vi "S101_temp_rise_red.vi"(0 "SI101_AverageReactorCoolantTemperature.lvclass":refnum<class "SI101_AverageReactorCoolantTemperature.lvclass">, 1 "3 JEC10 CT001B XQ01":dbl, 2 "3 JEC20 CT001B XQ01":dbl, 3 "3 JEC30 CT001B XQ01":dbl, 4 "3 JEC40 CT001B XQ01":dbl, 5 "error in (no error)":errorcluster, 6 "From Acquisition":T3, 8 "From SI100":T2) -> (12 "APs":cluster{"AP1":dbl, "AP2":dbl, "AP3":dbl}, 14 "SI101_AverageReactorCoolantTemperature.lvclass out":refnum<class "SI101_AverageReactorCoolantTemperature.lvclass">, 15 "ACT Loop 1":dbl, 16 "ACT Loop 2":dbl, 17 "ACT loop 3":dbl, 18 "ACT loop 4":dbl, 19 "error IO":errorcluster)   [LabVIEW 2022 SP3, in "SI101_AverageReactorCoolantTemperature.lvclass"]
uses:
  SI101_AverageReactorCoolantTemperature.lvclass
  SI101_AverageReactorCoolantTemperature.lvclass/SI101_AverageReactorCoolantTemperature.ctl
panel:
  in  "Set Params 4":T1
  in  "Set Params 3":T1
  in  "Set Params 2":T1
  in  "Set Params":T1
  # "SI101"
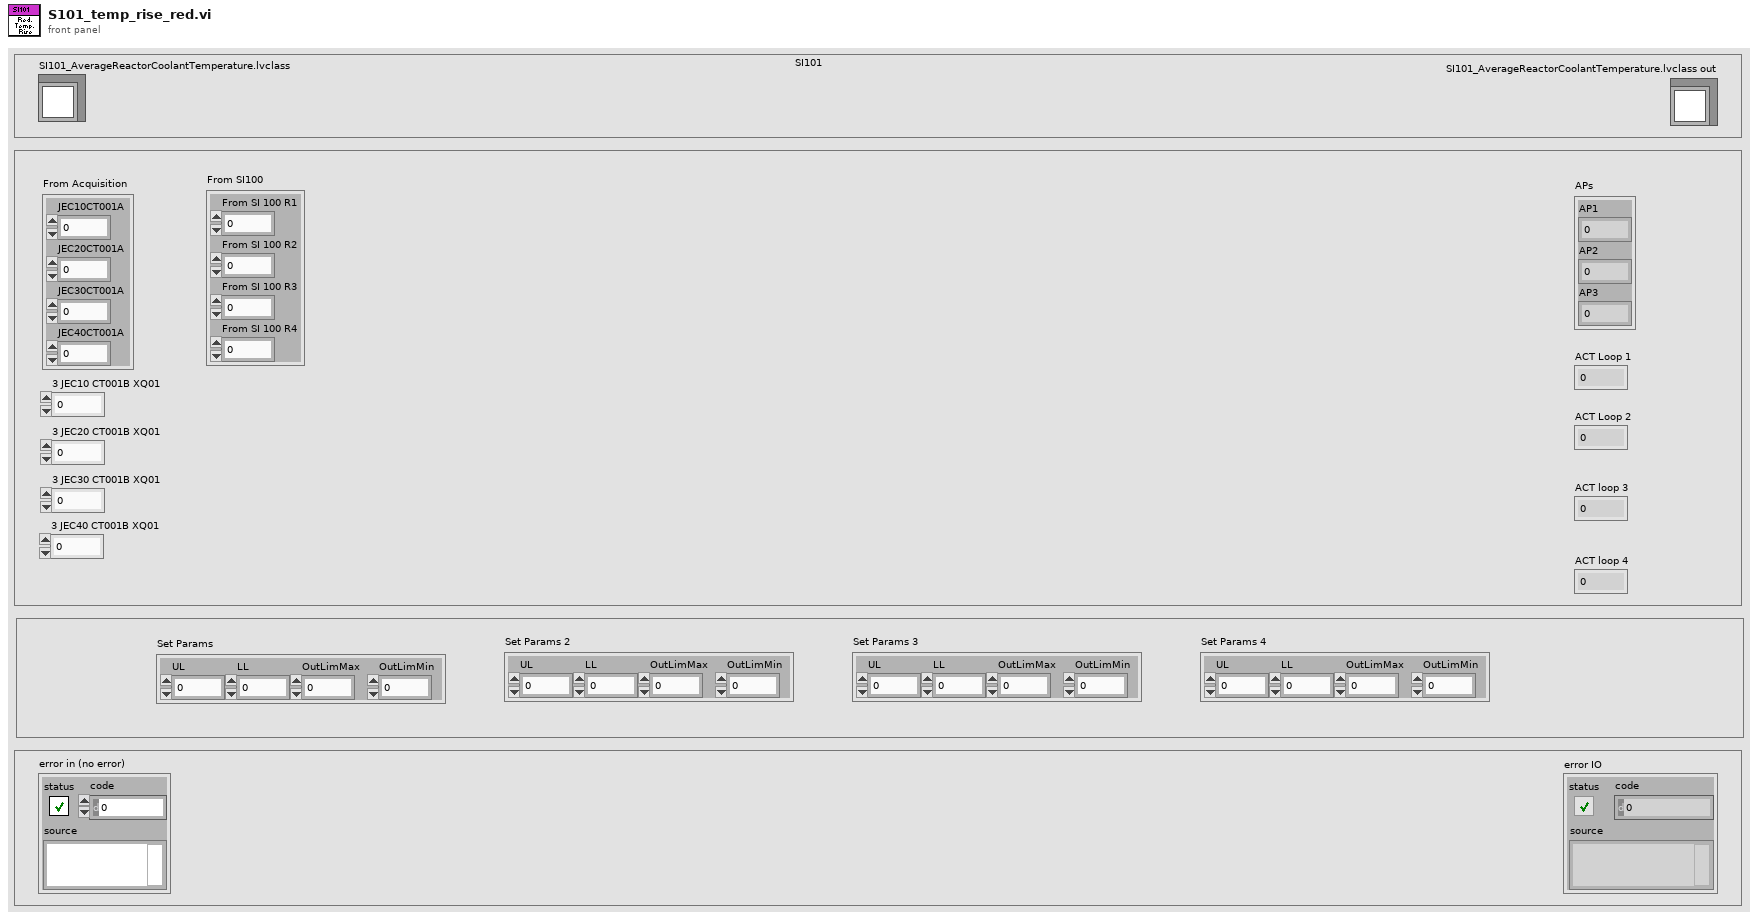
[diagram p1: front panel]
types:
  T1 = cluster{"UL":dbl, "LL":dbl, "OutLimMax":dbl, "OutLimMin":dbl}
  T2 = cluster{"From SI 100 R1":dbl, "From SI 100 R2":dbl, "From SI 100 R3":dbl, "From SI 100 R4":dbl}
  T3 = cluster{"JEC10CT001A":dbl, "JEC20CT001A":dbl, "JEC30CT001A":dbl, "JEC40CT001A":dbl}
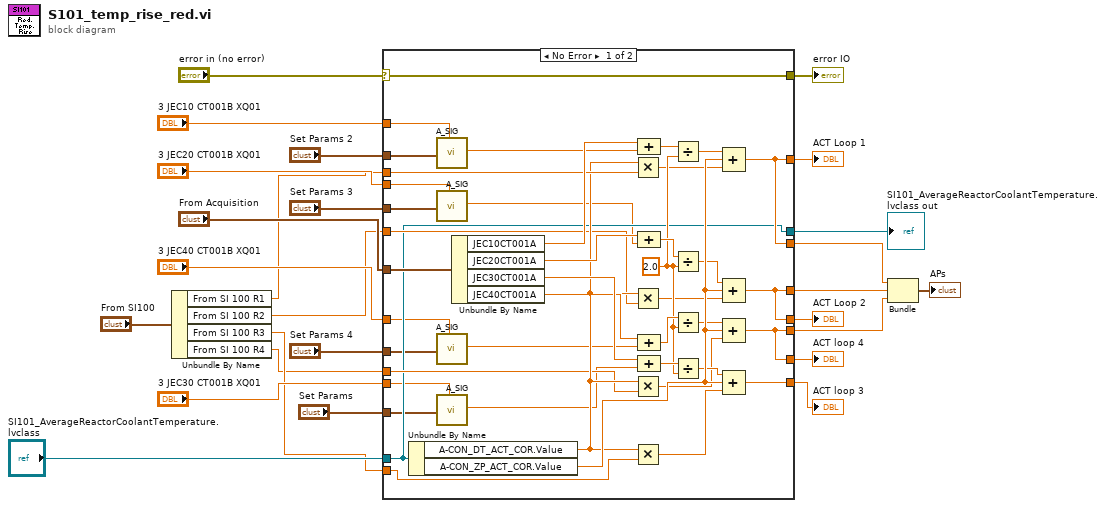
[diagram p0: block diagram]
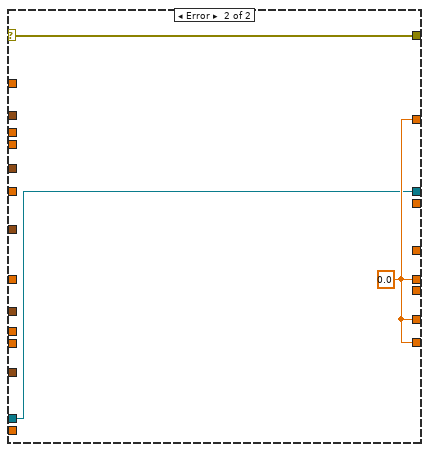
[diagram p2: hidden frame]
diagram:
  n1 = Unbundle By Name("From SI100") -> ("From SI 100 R1"=w13:dbl, "From SI 100 R2"=w12:dbl, "From SI 100 R3"=w11:dbl, "From SI 100 R4"=w10:dbl)
  n2 = case shown="No Error" "error in (no error)" {
    selector: "error in (no error)" -> [w68 w70]
    tunnel: [w42 w71] -> w25
    tunnel: [w41 w71] -> w24
    tunnel: [w43 w71] -> w23
    tunnel: [w40 w71] -> w22
    tunnel: [w68 w70] -> w21
    tunnel: "From Acquisition" -> [w67 _]
    tunnel: "3 JEC10 CT001B XQ01" -> [w35 _]
    tunnel: "3 JEC20 CT001B XQ01" -> [w33 _]
    tunnel: "3 JEC30 CT001B XQ01" -> [w38 _]
    tunnel: "3 JEC40 CT001B XQ01" -> [w31 _]
    tunnel: "SI101_AverageReactorCoolantTemperature.lvclass" -> [w39 w69]
    tunnel: w13 -> [w52 _]
    tunnel: w12 -> [w49 _]
    tunnel: w11 -> [w48 _]
    tunnel: w10 -> [w47 _]
    tunnel: [w42 _] -> w9
    tunnel: [w41 _] -> w8
    tunnel: [w40 _] -> w7
    tunnel: [w39 w69] -> w5
    tunnel: "Set Params" -> [w36 _]
    tunnel: "Set Params 2" -> [w29 _]
    tunnel: "Set Params 3" -> [w28 _]
    tunnel: "Set Params 4" -> [w27 _]
    frame No Error {
      w58 = 2.0
      n3 = Unbundle By Name(w39) -> ("A-CON_DT_ACT_COR.Value"=w50:dbl, "A-CON_ZP_ACT_COR.Value"=w56:dbl)
      n4 = call "A_SIG.vi"("Set Params"=w29, "Input"=w35) -> ("A_SIG_out"=w34:dbl)  [unwired: 16 in, 1 out]
      n5 = call "A_SIG.vi"("Set Params"=w28, "Input"=w33) -> ("A_SIG_out"=w32:dbl)  [unwired: 16 in, 1 out]
      n6 = call "A_SIG.vi"("Set Params"=w27, "Input"=w31) -> ("A_SIG_out"=w30:dbl)  [unwired: 16 in, 1 out]
      n7 = call "A_SIG.vi"("Set Params"=w36, "Input"=w38) -> ("A_SIG_out"=w37:dbl)  [unwired: 16 in, 1 out]
      n8 = Unbundle By Name(w67) -> ("JEC10CT001A"=w66:dbl, "JEC20CT001A"=w65:dbl, "JEC30CT001A"=w64:dbl, "JEC40CT001A"=w63:dbl)
      n9 = Multiply(x=w50, y=w52) -> (x*y=w51:dbl)
      n10 = Multiply(x=w50, y=w49) -> (x*y=w46:dbl)
      n11 = Multiply(x=w50, y=w47) -> (x*y=w44:dbl)
      n12 = Multiply(x=w50, y=w48) -> (x*y=w45:dbl)
      n13 = Compound Arithmetic op=ADD(w66, w34) -> (w62:dbl)
      n14 = Compound Arithmetic op=ADD(w65, w32) -> (w61:dbl)
      n15 = Compound Arithmetic op=ADD(w63, w30) -> (w59:dbl)
      n16 = Compound Arithmetic op=ADD(w64, w37) -> (w60:dbl)
      n17 = Divide(x=w62, y=w58) -> (x/y=w57:dbl)
      n18 = Divide(x=w61, y=w58) -> (x/y=w55:dbl)
      n19 = Divide(x=w59, y=w58) -> (x/y=w53:dbl)
      n20 = Divide(x=w60, y=w58) -> (x/y=w54:dbl)
      n21 = Compound Arithmetic op=ADD(w57, w56, w51) -> (w42:dbl)
      n22 = Compound Arithmetic op=ADD(w55, w56, w46) -> (w41:dbl)
      n23 = Compound Arithmetic op=ADD(w53, w56, w44) -> (w40:dbl)
      n24 = Compound Arithmetic op=ADD(w54, w56, w45) -> (w43:dbl)
    }
    frame Error {
      w71 = 0.0 ("ACT loop n")
    }
  }
  "ACT Loop 1" <- w25
  "ACT Loop 2" <- w24
  "ACT loop 3" <- w23
  "ACT loop 4" <- w22
  "error IO" <- w21
  "SI101_AverageReactorCoolantTemperature.lvclass out" <- w5
  n25 = Bundle(w9, w8, w7) -> (→"APs":cluster{dbl, dbl, dbl})  [unwired: 1 in]
